vi "Draw FPS.vi"(10 "Frame Rate":dbl, 11 "Screen in":picture) -> (3 "Screen out":picture)   [LabVIEW 2022 SP3, in "Application.lvlib"]
uses:
  Application.lvlib
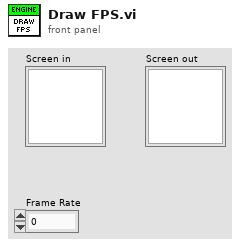
[diagram p1: front panel]
types:
  T1 = cluster{"horizontal":enum16{"left", "center", "right"}, "vertical":enum16{"top", "center", "bottom"}}
  T2 = enum16{"User-specified Font", "Application Font", "System Font", "Dialog Font"}
  T3 = cluster{"Font Name:":string, "Size":i16, "Strikeout?":bool, "Italic?":bool, "Underline?":bool, "Outline?":bool, "Shadow?":bool, "Bold?":bool}
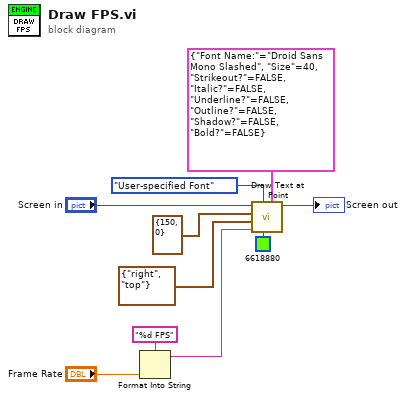
[diagram p0: block diagram]
diagram:
  n1 = Format Into String(format string="%d FPS", "Frame Rate") -> (resulting string=w8:string)  [unwired: 2 in, 1 out]
  n2 = call <vilib>:"Draw Text at Point.vi"("[user-specified font]"=T3 {"Font Name:"="Droid Sans Mono Slashed", "Size"=40, "Strikeout?"=FALSE, "Italic?"=FALSE, "Underline?"=FALSE, "Outline?"=FALSE, "Shadow?"=FALSE, "Bold?"=FALSE}, "text color(black)"=u32 6618880, "desired font(Application)"=T2."User-specified Font", "text"=w8, "alignment(left, top)"=T1 {"horizontal"=enum."right", "vertical"=enum."top"}, "origin"=cluster{"x":i16, "y":i16} {"x"=150, "y"=0}, "picture"="Screen in") -> ("new picture"=→"Screen out":picture)  [unwired: 3 in, 1 out]
